vi "GetReference.vi"(8 "error in":errorcluster, 11 "DiagramDisable in":refnum<class "DiagramDisable.lvclass">) -> (0 "error out":errorcluster, 1 "DDS reference":refnum<vi>, 3 "DiagramDisable out":refnum<class "DiagramDisable.lvclass">)   [LabVIEW 2014, in "Raspberry Pi Compatible Compiler for LabVIEW.lvlib" / "DiagramDisable.lvclass"]
uses:
  DiagramDisable.lvclass
  Generic/Generic.lvclass
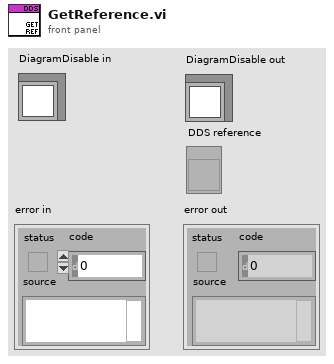
[diagram p1: front panel]
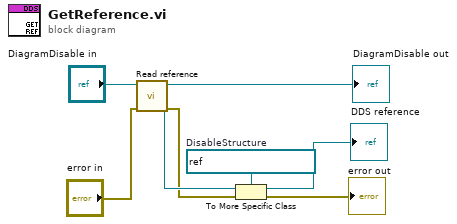
[diagram p0: block diagram]
diagram:
  w8 = refnum<vi> refnum  # DisableStructure
  n1 = call "Read reference.vi"("error in"="error in", "GObject in"="DiagramDisable in") -> ("error out"=w4:errorcluster, "reference"=w7:refnum<vi>, "GObject out"=→"DiagramDisable out":refnum<class "DiagramDisable.lvclass">)  [unwired: 5 in]
  n2 = To More Specific Class(target class=w8, reference=w7, error in=w4) -> (specific class reference=→"DDS reference":refnum<vi>, error out=→"error out":errorcluster)
